vi "WaitForMessage.vi"(0 "reference":refnum<class "VdTcpIP.lvclass">, 1 "MaxBytesToRead(10000)":i32=10000, 5 "error in (no error)":errorcluster, 7 "waitTime(-1=forever)":i32=-1) -> (14 "reference out":refnum<class "VdTcpIP.lvclass">, 15 "data out":string, 19 "error out":errorcluster)   [LabVIEW 2020, in "VdTcpIP.lvclass"]
doc: "Gets message from the listener connection"
uses:
  VdTcpIP.lvclass
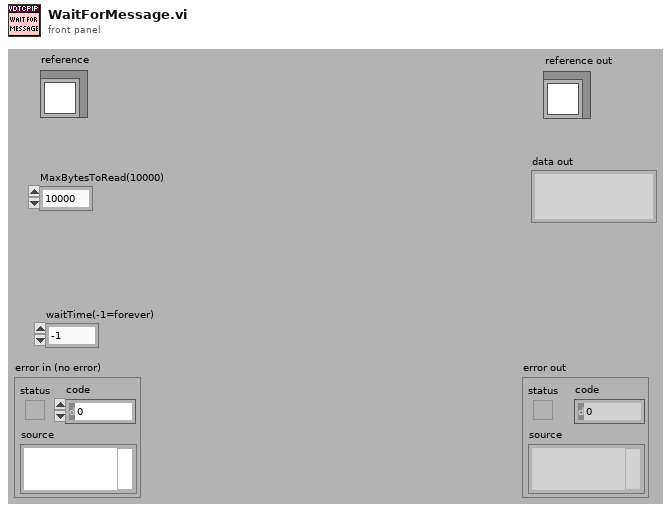
[diagram p1: front panel]
types:
  T1 = enum16{"Standard", "Buffered", "CRLF", "Immediate"}
  T2 = typedef "VdTcpIP.lvclass/ObjectAttributes.ctl" = cluster{"IP-Address":string, "Port":u16, "Connection":refnum<k5>, "Listener":refnum<k5>, "ListenerConnection":refnum<k5>, "Listner":bool, "ListnerProcessRunning":bool, "InConnections":refnum<k5>[], "InConnectionsIP":string[], "InConnectionAdded":refnum<notifier>, "RunVIOnNewConnection":variant, "DataToNewConnectionVI":cluster{"ControlName":string, "ControlValue":variant}[], "WebServicesURL_Location(http://...)":string, "WebServicesPostWebPage(*.asmx)":string, "Semaphore":T3, "AutoReConnectTimes":i32, "AutoReConnectInterval(ms)":i32, "ConnectionTimeout":i32}
  T3 = typedef "Semaphore RefNum" = refnum<k1>
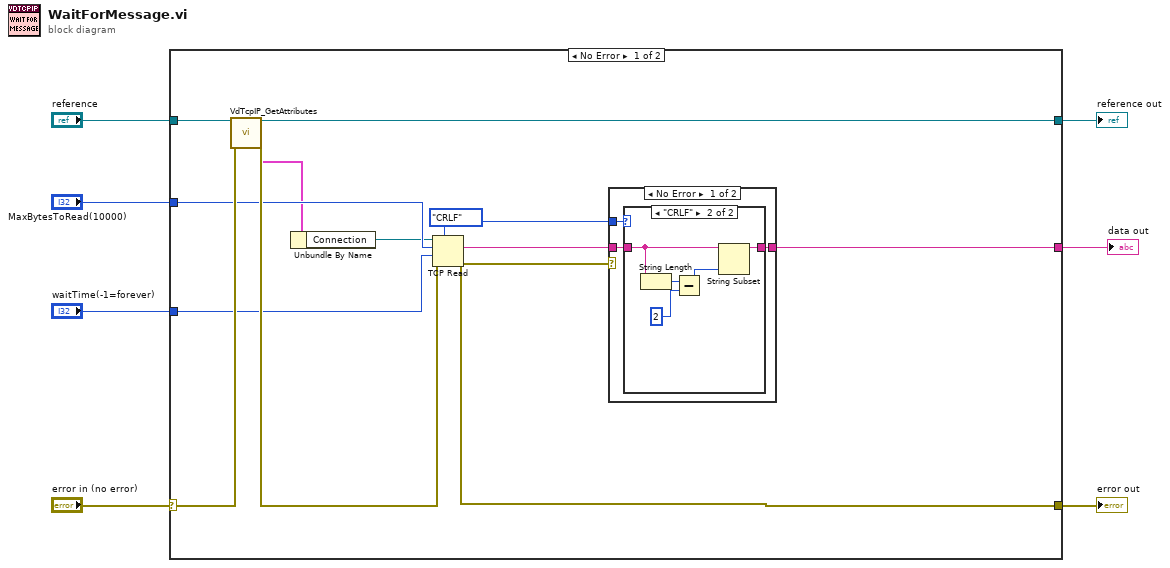
[diagram p0: block diagram]
diagram:
  n1 = case shown="No Error" "error in (no error)" {
    selector: "error in (no error)" -> [w19 w30]
    tunnel: "reference" -> [w18 w31]
    tunnel: [w10 w30] -> w5
    tunnel: [w9 w31] -> w4
    tunnel: "MaxBytesToRead(10000)" -> [w16 _]
    tunnel: "waitTime(-1=forever)" -> [w15 _]
    tunnel: [w13 _] -> w1
    frame No Error {
      w11 = T1."CRLF" ("mode (standard)")
      n2 = call "VdTcpIP_GetAttributes.vi"("reference in"=w18, "error in (no error)"=w19) -> ("reference out"=w9:refnum<class "VdTcpIP.lvclass">, "Data"=w8:T2, "error out"=w17:errorcluster)  [unwired: 1 in, 14 out]
      n3 = Unbundle By Name(w8) -> ("Connection"=w12:refnum<k5>)
      n4 = TCP Read(connection ID=w12, bytes to read=w16, error in (no error)=w17, 7:w11, 9:w15) -> (data out=w14:string, error out=w10:errorcluster)  [unwired: 1 out]
      n5 = case shown="No Error" w10 {
        tunnel: w14 -> [w21 w29]
        tunnel: w11 -> [w22 _]
        tunnel: [w20 w29] -> w13
        frame No Error {
          n6 = case shown="\"CRLF\"" w22 {
            tunnel: w21 -> [w23 w28]
            tunnel: [w23 w24] -> w20
            frame Default {
            }
            frame "CRLF" {
              n7 = String Length(string=w28) -> (length=w27:i32)
              n8 = Subtract(x=w27, y=2) -> (x-y=w25:i32)
              n9 = String Subset(string=w28, length (rest)=w25) -> (substring=w24:string)  [unwired: 1 out]
            }
          }
        }
        frame Error {
        }
      }
    }
    frame Error {
    }
  }
  "reference out" <- w4
  "error out" <- w5
  "data out" <- w1
